vi "Run Stimulus Profile Session.vi"(8 "error in (no error)":errorcluster, 11 "Session Ref in":T1) -> (0 "error out":errorcluster, 3 "Session Ref out":T1)   [LabVIEW 2020, in "NI_VS Sequence Execution Interface.lvlib"]
doc: "Runs all sequences in an NI VeriStand stimulus profile session."
uses:
  <vilib>/NI VeriStand/Execution/SequenceExecutionInterface/NI_VS Sequence Execution Interface.lvlib
  <vilib>/NI VeriStand/Execution/SequenceExecutionInterface/Stimulus Profile Session Ref.ctl
  NationalInstruments.VeriStand.ClientAPI
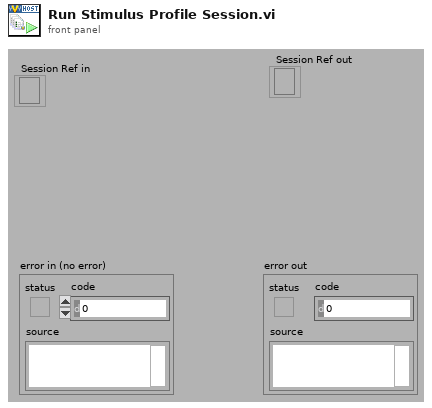
[diagram p1: front panel]
types:
  T1 = typedef "NI_VS Sequence Execution Interface.lvlib/Stimulus Profile Session Ref.ctl" = refnum<k24>
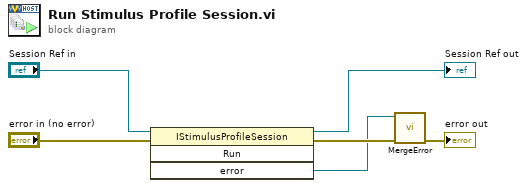
[diagram p0: block diagram]
diagram:
  n1 = invoke class="IStimulusProfileSession" method="Run"(reference="Session Ref in", error in="error in (no error)") -> (reference out=→"Session Ref out":T1, error out=w3:errorcluster, "error"=w2:refnum<k24>)  [unwired: 2 in, 1 out]
  n2 = call <vilib>:"MergeError.vi"("error in (no error)"=w3, "Error"=w2) -> ("error out"=→"error out":errorcluster)  [unwired: 9 out]
